vi "x_y_plot_live.vi"() -> ()   [LabVIEW 2020]
panel:
  in  "Boolean":bool
  out "XY Graph":cluster{i32[], i32[]}(graph)
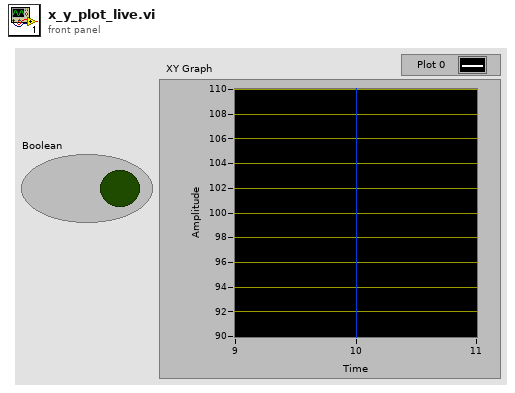
[diagram p1: front panel]
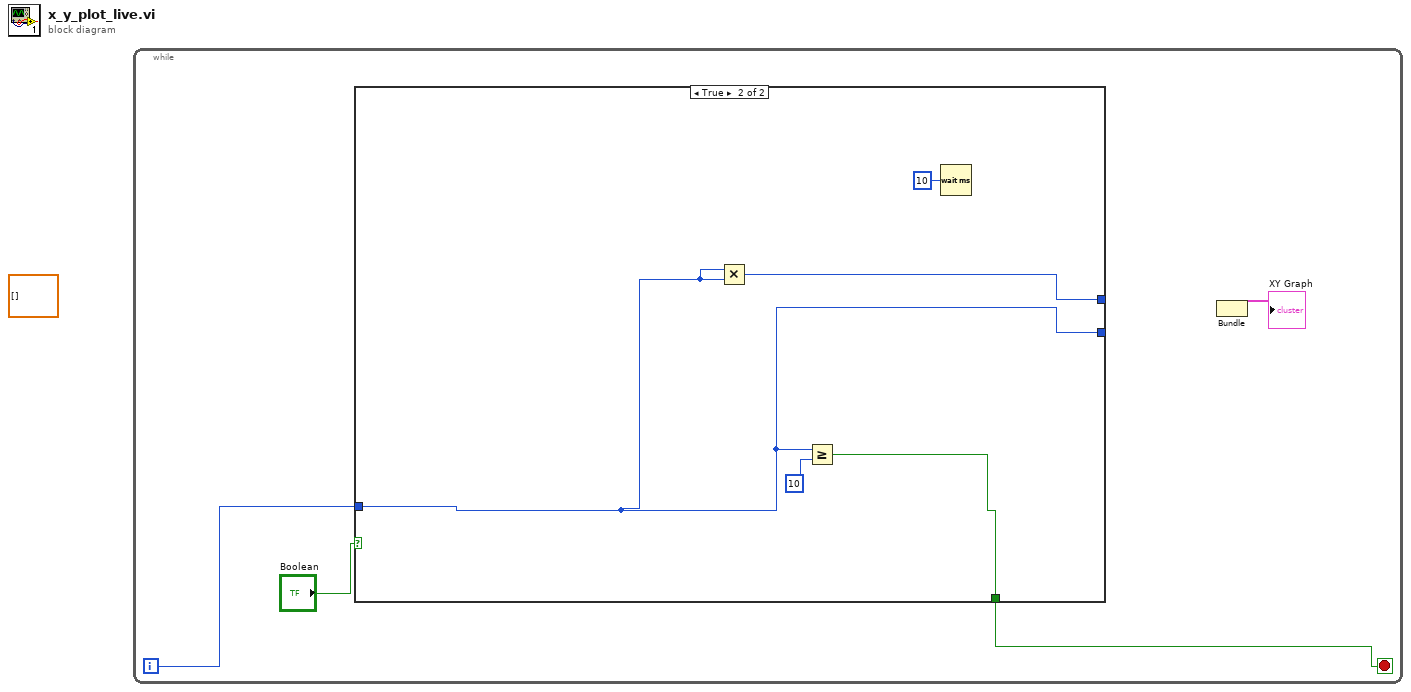
[diagram p0: block diagram]
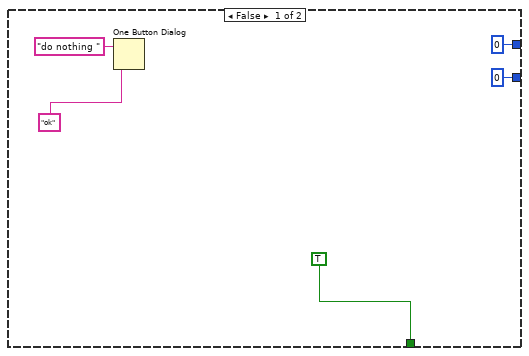
[diagram p2: hidden frame]
diagram:
  (unwired) dbl[] []
  n1 = while {
    i -> [w2]
    stop <- w1 stop-if-true
    n2 = case shown="True" "Boolean" {
      tunnel: [0 w14] -> w6
      tunnel: [0 w17] -> _
      tunnel: w2 -> [_ w14]
      tunnel: [TRUE w13] -> w1
      frame False {
        n3 = One Button Dialog(message="do nothing ", button name ("OK")="ok") -> ()  [unwired: 1 out]
      }
      frame True {
        n4 = Multiply(x=w14, y=w14) -> (x*y=w17:i32)
        n5 = Greater Or Equal?(x=w14, y=10) -> (x >= y?=w13:bool)
        n6 = Wait (ms)(milliseconds to wait=u32 10) -> ()  [unwired: 1 out]
      }
    }
    n7 = Bundle() -> (→"XY Graph":cluster{void, void}, w4, w3)  [unwired: 1 in]
  }
